vi "Set IPS PSU Targets.vi"(8 "error in (no error)":errorcluster, 9 "Target Field Rate (T/min)":dbl format="%#.2f", 10 "Target Field (T)":dbl format="%#.2f", 11 "Instrument.Oxford1820 in":refnum<class "Instrument.Oxford1820.lvclass">) -> (0 "error out":errorcluster, 2 "Response":string, 3 "Instrument.Oxford1820 out":refnum<class "Instrument.Oxford1820.lvclass">)   [LabVIEW 2019, in "Instrument.Oxford1820.lvclass"]
uses:
  Instrument.Oxford1820.lvclass
  Instrument.Oxford1820.lvclass/Instrument.Oxford1820.ctl
  <instrlib>/Mercury iXX/Public/Libraries/Magnet/Open/Open Magnet Device.vi
  <instrlib>/Mercury iXX/Public/Libraries/Magnet/Signals/Set/Target Field Rate (Set).vi
  <instrlib>/Mercury iXX/Public/Libraries/Magnet/Signals/Set/Target Field (Set).vi
  <instrlib>/Mercury iXX/Public/Libraries/Magnet/Signals/Read/Target Field Rate (Read).vi
  <instrlib>/Mercury iXX/Public/Libraries/Magnet/Signals/Read/Target Field (Read).vi
  <instrlib>/Mercury iXX/Mercury iXX.lvlib
  <instrlib>/Mercury iXX/Public/Libraries/Magnet.lvlib
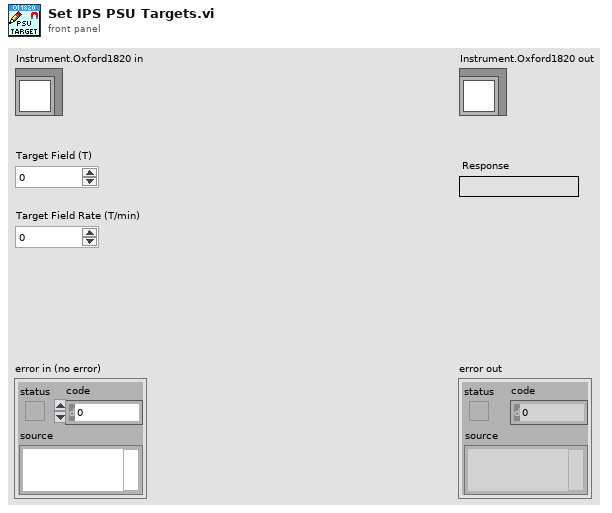
[diagram p1: front panel]
types:
  T1 = typedef "Mercury iXX.lvlib/Mercury Reference.ctl" = cluster{"Comms":refnum<visa-resource-name>, "Device ID":string[], "Comms Layer":T2, "Command":string, "Query reference":T3}
  T2 = typedef "Mercury iXX.lvlib/Comms Transport Layer.ctl" = enum16{"Ethernet TCP/IP", "USB", "ISOBus - RS-232", "GPIB"}
  T3 = typedef "Mercury iXX.lvlib/Query Dynamic Reference.ctl" = refnum<vi>
  T4 = typedef "Mercury iXX.lvlib/Response String.ctl" = string
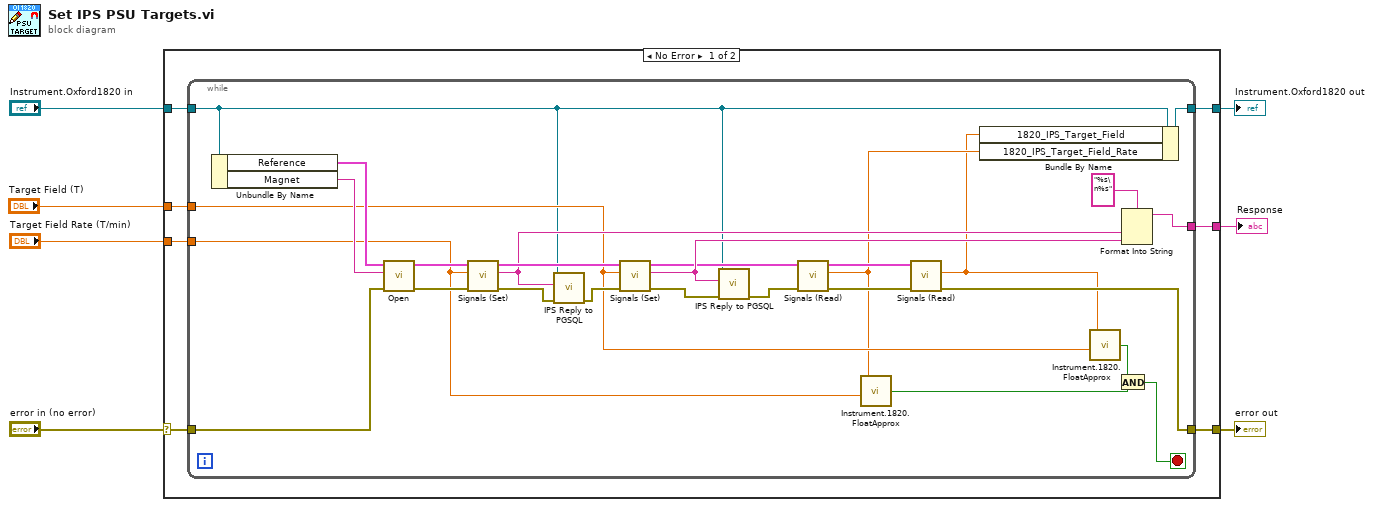
[diagram p0: block diagram]
diagram:
  n1 = case shown="No Error" "error in (no error)" {
    selector: "error in (no error)" -> [w13 w43]
    tunnel: [w9 w43] -> w6
    tunnel: [w8 w42] -> w4
    tunnel: "Instrument.Oxford1820 in" -> [w14 w42]
    tunnel: [w10 _] -> w3
    tunnel: "Target Field (T)" -> [w12 _]
    tunnel: "Target Field Rate (T/min)" -> [w11 _]
    frame No Error {
      n2 = while {
        tunnel: w14 -> [w17]
        tunnel: w13 -> [w40]
        tunnel: w12 -> [w19]
        tunnel: w11 -> [w20]
        tunnel: [w30] -> w10
        tunnel: [w24] -> w9
        tunnel: [w18] -> w8
        stop <- w21 stop-if-true
        n3 = Unbundle By Name(w17) -> ("Reference"=w41:T1, "Magnet"=w25:string)
        n4 = call-poly <instrlib>:"Open.vi"("error in (no error)"=w40, "Device Identifier"=w25, "Mercury Reference In"=w41) -> ("error out"=w34:errorcluster, "Mercury Reference Out"=w35:T1)  [unwired: 7 out]
        n5 = call-poly <instrlib>:"Signals (Set).vi"("error in"=w34, "Target Field Rate"=w20, "Mercury Reference In"=w35) -> ("error out"=w38:errorcluster, "Response"=w31:T4, "Mercury Reference Out"=w36:T1)  [unwired: 2 in, 4 out]
        n6 = call "IPS Reply to PGSQL.vi"("error in (no error)"=w38, "Response"=w31, "Instrument.1820 in"=w17) -> ("error out"=w37:errorcluster)  [unwired: 7 in, 1 out]
        n7 = call-poly <instrlib>:"Signals (Set).vi"("error in"=w37, "Target Field"=w19, "Mercury Reference In"=w36) -> ("error out"=w39:errorcluster, "Response"=w32:T4, "Mercury Reference Out"=w28:T1)  [unwired: 2 in, 4 out]
        n8 = call "IPS Reply to PGSQL.vi"("error in (no error)"=w39, "Response"=w32, "Instrument.1820 in"=w17) -> ("error out"=w29:errorcluster)  [unwired: 7 in, 1 out]
        n9 = call-poly <instrlib>:"Signals (Read).vi"("error in"=w29, "Mercury Reference In"=w28) -> ("error out"=w26:errorcluster, "Target Field Rate"=w16:dbl, "Mercury Reference Out"=w27:T1)  [unwired: 5 in, 2 out]
        n10 = call "Instrument.1820.FloatApprox.vi"("y"=w20, "x"=w16) -> ("x ~ y?"=w22:bool)  [unwired: 4 in]
        n11 = call-poly <instrlib>:"Signals (Read).vi"("error in"=w26, "Mercury Reference In"=w27) -> ("error out"=w24:errorcluster, "Target Field"=w15:dbl)  [unwired: 5 in, 3 out]
        n12 = Bundle By Name(cluster=w17, "1820_IPS_Target_Field"=w15, "1820_IPS_Target_Field_Rate"=w16) -> (w18:refnum<class "Instrument.Oxford1820.lvclass">)
        n13 = call "Instrument.1820.FloatApprox.vi"("y"=w19, "x"=w15) -> ("x ~ y?"=w23:bool)  [unwired: 4 in]
        n14 = And(x=w23, y=w22) -> (x .and. y?=w21:bool)
        n15 = Format Into String(format string="%s\n%s", w31, w32) -> (resulting string=w30:string)  [unwired: 2 in, 1 out]
      }
    }
    frame Error {
    }
  }
  "error out" <- w6
  "Instrument.Oxford1820 out" <- w4
  "Response" <- w3
